vi "tcpcontrol.vi"() -> ()   [LabVIEW 2018]
uses:
  Downloads/sabertooth-packetized-control-master/sabertooth-packetized-control-master/code/package/controls/Sabertooth Baud Rate Select.ctl
  <vilib>/myRIO/Instrument Drivers/Onboard IO/DIO/typedefs/DIO Reference.ctl
  <vilib>/myRIO/Common/Instrument Driver Framework/Utilities/typedefs/myRIO Generic Hardware Reference.ctl
  <vilib>/myRIO/Common/Instrument Driver Framework/Utilities/typedefs/Hardware Version Enum.ctl
  <vilib>/myRIO/Common/Instrument Driver Framework/Utilities/typedefs/myRIO v1.0 Reference.ctl
  <vilib>/myRIO/Common/Instrument Driver Framework/Utilities/typedefs/Generic FPGA Reference.ctl
  <vilib>/myRIO/Common/Instrument Driver Framework/myRIO v1.0/DIO/typedefs/DIO Channels List.ctl
  <vilib>/myRIO/Common/Instrument Driver Framework/myRIO v1.0/DIO/typedefs/DIO Channels Enum.ctl
  <vilib>/userdefined/High Color/nirio_resource_hc.ctl
  <vilib>/myRIO/Common/Instrument Driver Framework/Utilities/vis/Is FPGA Ref Available.vi
  <vilib>/myRIO/Common/Instrument Driver Framework/myRIO v1.0/DIO/vis/myRIO v1.1 Open DIO.vi
  <vilib>/myRIO/Instrument Drivers/Onboard IO/DIO/vis/Write.vi
  <vilib>/myRIO/Common/Instrument Driver Framework/Utilities/vis/Validate Channels.vi
  <vilib>/myRIO/Common/Instrument Driver Framework/myRIO v1.0/DIO/vis/myRIO v1.0 Reserve DIO.vi
  <vilib>/myRIO/Common/Instrument Driver Framework/myRIO v1.0/Resource Manager/vis/myRIO v1.0 Reserve Channel List.vi
  <vilib>/myRIO/Common/Instrument Driver Framework/myRIO v1.0/DIO/vis/myRIO v1.0 Build MUX Configuration DIO.vi
  <vilib>/myRIO/Common/Instrument Driver Framework/myRIO v1.0/Resource Manager/vis/myRIO v1.0 Reserve Channel.vi
  <vilib>/myRIO/Common/Instrument Driver Framework/myRIO v1.0/Resource Manager/vis/myRIO v1.0 Unreserve Channel.vi
  <vilib>/myRIO/Common/Instrument Driver Framework/myRIO v1.0/Resource Manager/vis/myRIO v1.0 Create Configuration List.vi
  <vilib>/myRIO/Common/Instrument Driver Framework/myRIO v1.0/Resource Manager/vis/myRIO v1.0 Build Mutex Name.vi
  <vilib>/Instr/_visa.llb/VISA Configure Serial Port (Instr).vi
  <vilib>/Utility/VariantDataType/GetNumericInfo.vi
  <vilib>/Utility/error.llb/Error Cluster From Error Code.vi
  <vilib>/myRIO/Common/Instrument Driver Framework/myRIO v1.0/myRIO v1.1 Open.vi
  <vilib>/myRIO/Common/Instrument Driver Framework/Utilities/vis/IO Manager.vi
  <vilib>/myRIO/Common/Instrument Driver Framework/Utilities/vis/Configuration Manager.vi
  <vilib>/myRIO/Common/Instrument Driver Framework/myRIO v1.0/Resource Manager/vis/myRIO v1.0 Configure IO.vi
  <vilib>/myRIO/Common/Instrument Driver Framework/myRIO v1.0/myRIO v1.0 Close.vi
  <vilib>/myRIO/Common/Instrument Driver Framework/myRIO v1.0/DIO/vis/myRIO v1.0 Write DIO.vi
  <vilib>/myRIO/Express VI/Onboard Devices/LED/LED Express VI.xnode
  <vilib>/myRIO/Instrument Drivers/Onboard IO/DIO/vis/myRIO DIO Open.xnode
  <vilib>/myRIO/Instrument Drivers/Onboard IO/DIO/DIO.lvlib
panel:
  in  "stop 2":bool
  in  "Current Baud Rate":T1=115200 items=["2400 baud"=2400, "9600 baud"=9600, "19200 baud"=19200, "38400 baud"=38400, "115200 baud"=115200]
  in  "stop":bool
  out "Loop Time":u32
  out "error out":errorcluster
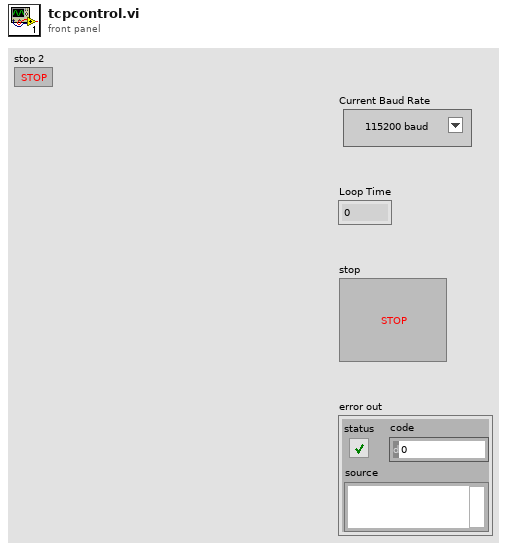
[diagram p1: front panel]
types:
  T1 = typedef "Sabertooth Baud Rate Select.ctl" = u32
  T2 = typedef "DIO.lvlib/DIO Reference.ctl" = cluster{"myRIO Reference":T3, "DIO Channels List":T7}
  T3 = typedef "myRIO Generic Hardware Reference.ctl" = cluster{"myRIO Model":T4, "myRIO Hardware Reference":T5}
  T4 = typedef "Hardware Version Enum.ctl" = enum16{"Unknown", "myRIO-1900", "myRIO-1950", "roboRIO", "NI ELVIS RIO CM", "ELVIS III"}
  T5 = typedef "myRIO v1.0 Reference.ctl" = cluster{"Generic FPGA Reference":T6, "Allow multiple opens":bool}
  T6 = typedef "Generic FPGA Reference.ctl" = refnum<k20>
  T7 = typedef "DIO Channels List.ctl" = T8[]
  T8 = typedef "DIO Channels Enum.ctl" = enum16{"Not Connected", "C/DIO0", "C/DIO1", "C/DIO2", "C/DIO3", "C/DIO4", "C/DIO5", "C/DIO6", "C/DIO7", "A/DIO0", "A/DIO1", "A/DIO2", "A/DIO3", "A/DIO4", "A/DIO5", "A/DIO6", "A/DIO7", "A/DIO8", "A/DIO9", "A/DIO10", "A/DIO11", "A/DIO12", "A/DIO13", "A/DIO14", "A/DIO15", "A/DIO16", "A/DIO17", "A/DIO18", "A/DIO19", "B/DIO0", "B/DIO1", "B/DIO2", "B/DIO3", "B/DIO4", "B/DIO5", "B/DIO6", "B/DIO7", "B/DIO8", "B/DIO9", "B/DIO10", "B/DIO11", "B/DIO12", "B/DIO13", "B/DIO14", "B/DIO15", "B/DIO16", "B/DIO17", "B/DIO18", "B/DIO19", "LED0", "LED1", "LED2", "LED3", "Button0", "DIO/DIO0", "DIO/DIO1", "DIO/DIO2", "DIO/DIO3", "DIO/DIO4", "DIO/DIO5", "DIO/DIO6", "DIO/DIO7", "DIO/DIO8", "DIO/DIO9", "SPI/CS0", "SPI/CS1", "SPI/CS2", "SPI/CS3", "LED RADIO (Green)", "LED RADIO (Red)", "LED COMM (Green)", "LED COMM (Red)", "LED MODE (Green)", "LED MODE (Red)"}
  T9 = typedef "nirio_resource_hc.ctl" = tag
  T10 = enum16{"Standard", "Buffered", "CRLF", "Immediate"}
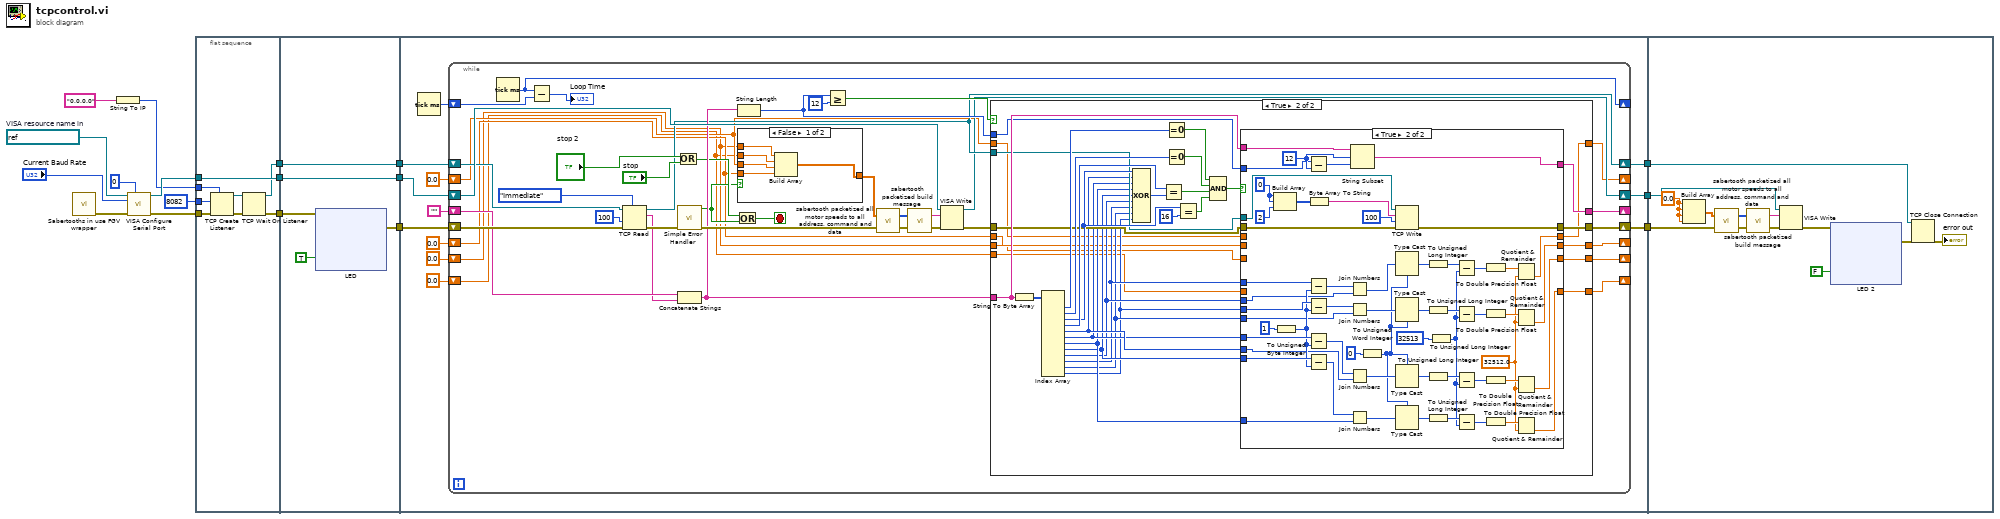
[diagram p0: block diagram]
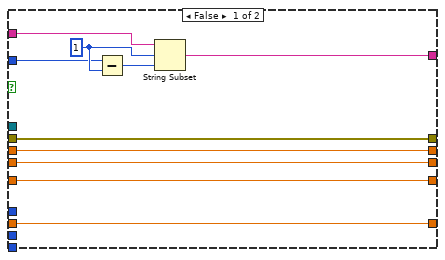
[diagram p3: hidden frame]
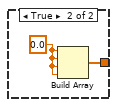
[diagram p4: hidden frame]
diagram:
  w18 = refnum<visa-resource-name> "ASRL1::INSTR"  # VISA resource name in
  n1 = call "Sabertooths in use FGV wrapper.vi"() -> ("error out"=w15:errorcluster)  [unwired: 11 in]
  n2 = String To IP(1:"0.0.0.0") -> (0:w12:u32)
  n3 = call-poly "VISA Configure Serial Port"("VISA resource name"=w18, "timeout (10sec)"=u32 0, "baud rate (9600)"="Current Baud Rate", "error in (no error)"=w15) -> ("VISA resource name out"=w17:refnum<visa-resource-name>, "error out"=w11:errorcluster)  [unwired: 10 in]
  n4 = flat-sequence {
    tunnel: w17 -> [w26]
    tunnel: [w26] -> w9
    tunnel: [w25] -> w7
    tunnel: [w24] -> w5
    tunnel: w12 -> [w23]
    tunnel: w11 -> [w22]
    tunnel: u16 8082 ("port") -> [w21]
    tunnel: w9 -> [w31]
    tunnel: [w31] -> w8
    tunnel: w7 -> [w29]
    tunnel: [w28] -> w6
    tunnel: w5 -> [w30]
    tunnel: [w30] -> w4
    tunnel: w8 -> [w78]
    tunnel: w6 -> [w76]
    tunnel: w4 -> [w75]
    tunnel: [w69] -> w3
    tunnel: [w68] -> w2
    tunnel: [w67] -> w1
    tunnel: w3 -> [w234]
    tunnel: w2 -> [w237]
    tunnel: w1 -> [w231]
    frame #0 {
      n5 = TCP Create Listener(7:w23, 8:w22, 10:w21) -> (0:w20:errorcluster, 3:w19:refnum<k5>)  [unwired: 2 in, 1 out]
      n6 = TCP Wait On Listener(8:w20, 11:w19) -> (0:w25:errorcluster, 3:w24:refnum<k5>)  [unwired: 2 in, 3 out]
    }
    frame #1 {
      n7 = xnode "LED"("LED0"=TRUE, "error in (no error)"=w29) -> ("error out"=w28:errorcluster)
    }
    frame #2 {
      n8 = Tick Count (ms)() -> (millisecond timer value=w77:u32)
      n9 = while {
        shift-right: [w114] -> _
        shift-left: w77 -> [w116]
        shift-right: [w90] -> w67
        shift-left: w75 -> [w107]
        shift-right: [w95] -> _
        shift-left: "" -> [w100]
        shift-right: [w86] -> _
        shift-left: 0.0 -> [w79]
        shift-right: [w85] -> _
        shift-left: 0.0 -> [w82]
        shift-right: [w84] -> _
        shift-left: 0.0 -> [w80]
        shift-right: [w83] -> _
        shift-left: 0.0 -> [w81]
        shift-right: [w88] -> w69
        shift-left: w76 -> [w106]
        shift-right: [w87] -> w68
        shift-left: w78 -> [w117]
        stop <- w92 stop-if-true
        n10 = Tick Count (ms)() -> (millisecond timer value=w114:u32)
        n11 = Subtract(x=w114, y=w116) -> (x-y=→"Loop Time":u32)
        n12 = TCP Read(connection ID=w107, error in (no error)=w106, 7:T10."Immediate" ("mode (standard)"), 9:100) -> (connection ID out=w90:refnum<k5>, data out=w99:string, error out=w104:errorcluster)  [unwired: 1 in]
        n13 = Or(x="stop 2", y="stop") -> (x .or. y?=w94:bool)
        n14 = call <vilib>:"Simple Error Handler.vi"("error in (no error)"=w104) -> ("error?"=w93:bool, "error out"=w103:errorcluster)  [unwired: 4 in, 3 out]
        n15 = Concatenate Strings(w100, w99) -> (w96:string)
        n16 = Or(x=w94, y=w93) -> (x .or. y?=w92:bool)
        n17 = String Length(string=w96) -> (length=w91:i32)
        n18 = case shown="False" w93 {
          tunnel: [w224 w229] -> w102
          tunnel: w80 -> [w228 _]
          tunnel: w79 -> [w227 _]
          tunnel: w81 -> [w226 _]
          tunnel: w82 -> [w225 _]
          frame False {
            n19 = Build Array(w228, w227, w226, w225) -> (w224:dbl[])
          }
          frame True {
            w230 = 0.0
            n20 = Build Array(w230, w230, w230, w230) -> (w229:dbl[])
          }
        }
        n21 = Greater Or Equal?(x=w91, y=12) -> (x >= y?=w97:bool)
        n22 = call "sabertooth packetized all motor speeds to all address, command and data.vi"("error in (no error)"=w103, "All Motor Speeds"=w102) -> ("error out"=w112:errorcluster, "Data to write"=w113:u8[][][])
        n23 = call "sabertooth packetized build message.vi"("error in (no error)"=w112, "Data to write"=w113) -> ("error out"=w111:errorcluster, "Uart Write Data"=w110:string)
        n24 = VISA Write(VISA resource name=w117, write buffer=w110, error in (no error)=w111) -> (VISA resource name out=w87:refnum<visa-resource-name>, error out=w89:errorcluster)  [unwired: 1 out]
        n25 = case shown="True" w97 {
          tunnel: w96 -> [w123 w145]
          tunnel: [w123 w144] -> w95
          tunnel: w91 -> [_ w143]
          tunnel: w90 -> [_ w142]
          tunnel: w89 -> [w122 w141]
          tunnel: [w122 w140] -> w88
          tunnel: [w118 w131] -> w86
          tunnel: [w121 w130] -> w85
          tunnel: [w119 w129] -> w84
          tunnel: [w120 w128] -> w83
          tunnel: w82 -> [w121 w127]
          tunnel: w81 -> [w120 w126]
          tunnel: w80 -> [w119 w125]
          tunnel: w79 -> [w118 w124]
          frame False {
          }
          frame True {
            n26 = String To Byte Array(string=w145) -> (unsigned byte array=w157:u8[])
            n27 = Index Array(array=w157) -> (element #1=w156:u8, element #2=w155:u8, element #3=w148:u8, element #4=w154:u8, element #5=w139:u8, element #6=w138:u8, element #7=w137:u8, element #8=w136:u8, element #9=w135:u8, element #10=w134:u8, element #11=w133:u8, element #12=w132:u8)  [unwired: 12 in]
            n28 = Compound Arithmetic op=XOR(w148, w139, w138, w137, w136, w135, w134, w133, w132) -> (w153:u8)
            n29 = Equal?(x=w154, y=w153) -> (x = y?=w150:bool)
            n30 = Equal To 0?(x=w156) -> (x = 0?=w152:bool)
            n31 = Equal To 0?(x=w155) -> (x = 0?=w151:bool)
            n32 = Equal?(x=w148, y=16) -> (x = y?=w149:bool)
            n33 = Compound Arithmetic op=AND(w152, w151, w150, w149) -> (w146:bool)
            n34 = case shown="True" w146 {
              tunnel: w145 -> [w164 w221]
              tunnel: [w163 w220] -> w144
              tunnel: w143 -> [w165 w219]
              tunnel: w142 -> [_ w212]
              tunnel: w141 -> [w162 w214]
              tunnel: [w162 w213] -> w140
              tunnel: w139 -> [_ w171]
              tunnel: w138 -> [_ w205]
              tunnel: w137 -> [_ w169]
              tunnel: w136 -> [_ w199]
              tunnel: w135 -> [_ w175]
              tunnel: w134 -> [_ w190]
              tunnel: w133 -> [_ w173]
              tunnel: w132 -> [_ w184]
              tunnel: [w158 w183] -> w131
              tunnel: [w161 w182] -> w130
              tunnel: [w159 w181] -> w129
              tunnel: [w160 w180] -> w128
              tunnel: w127 -> [w161 _]
              tunnel: w126 -> [w160 _]
              tunnel: w125 -> [w159 _]
              tunnel: w124 -> [w158 _]
              frame False {
                w166 = 1
                n35 = Subtract(x=w165, y=w166) -> (x-y=w167:i32)
                n36 = String Subset(string=w164, offset (0)=w166, length (rest)=w167) -> (substring=w163:string)
              }
              frame True {
                w176 = 32512.0
                w218 = 0
                w222 = 12
                n37 = Build Array(w218, w218, 2) -> (w216:i32[])
                n38 = To Unsigned Byte Integer(number=1) -> (unsigned 8bit integer=w178:u8)
                n39 = Subtract(x=w219, y=w222) -> (x-y=w223:i32)
                n40 = Subtract(x=w190, y=w178) -> (x-y=w174:u8)
                n41 = Subtract(x=w184, y=w178) -> (x-y=w172:u8)
                n42 = Subtract(x=w205, y=w178) -> (x-y=w170:u8)
                n43 = Subtract(x=w199, y=w178) -> (x-y=w168:u8)
                n44 = Byte Array To String(unsigned byte array=w216) -> (string=w215:string)
                n45 = Join Numbers(hi=w174, lo=w175) -> ((hi.lo)=w198:u16)
                n46 = Join Numbers(hi=w172, lo=w173) -> ((hi.lo)=w189:u16)
                n47 = Join Numbers(hi=w170, lo=w171) -> ((hi.lo)=w210:u16)
                n48 = Join Numbers(hi=w168, lo=w169) -> ((hi.lo)=w204:u16)
                n49 = String Subset(string=w221, offset (0)=w222, length (rest)=w223) -> (substring=w220:string)
                n50 = To Unsigned Word Integer(number=0) -> (unsigned 16bit integer=w179:u16)
                n51 = TCP Write(connection ID=w212, data in=w215, error in (no error)=w214, 9:100) -> (error out=w213:errorcluster)  [unwired: 2 out]
                n52 = Type Cast(type=w179, x=w198) -> (*(type *) &x=w195:u16)
                n53 = Type Cast(type=w179, x=w189) -> (*(type *) &x=w188:u16)
                n54 = Type Cast(type=w179, x=w210) -> (*(type *) &x=w209:u16)
                n55 = Type Cast(type=w179, x=w204) -> (*(type *) &x=w203:u16)
                n56 = To Unsigned Long Integer(number=w195) -> (unsigned 32bit integer=w194:u32)
                n57 = To Unsigned Long Integer(number=w188) -> (unsigned 32bit integer=w187:u32)
                n58 = To Unsigned Long Integer(number=w209) -> (unsigned 32bit integer=w208:u32)
                n59 = To Unsigned Long Integer(number=w203) -> (unsigned 32bit integer=w202:u32)
                n60 = To Unsigned Long Integer(number=32513) -> (unsigned 32bit integer=w177:u32)
                n61 = Subtract(x=w194, y=w177) -> (x-y=w191:u32)
                n62 = Subtract(x=w187, y=w177) -> (x-y=w185:u32)
                n63 = Subtract(x=w208, y=w177) -> (x-y=w206:u32)
                n64 = Subtract(x=w202, y=w177) -> (x-y=w200:u32)
                n65 = To Double Precision Float(number=w191) -> (double precision float=w192:dbl)
                n66 = To Double Precision Float(number=w185) -> (double precision float=w186:dbl)
                n67 = To Double Precision Float(number=w206) -> (double precision float=w207:dbl)
                n68 = To Double Precision Float(number=w200) -> (double precision float=w201:dbl)
                n69 = Quotient & Remainder(x=w192, y=w176) -> (floor(x/y)=w180:dbl)  [unwired: 1 out]
                n70 = Quotient & Remainder(x=w186, y=w176) -> (floor(x/y)=w182:dbl)  [unwired: 1 out]
                n71 = Quotient & Remainder(x=w207, y=w176) -> (floor(x/y)=w181:dbl)  [unwired: 1 out]
                n72 = Quotient & Remainder(x=w201, y=w176) -> (floor(x/y)=w183:dbl)  [unwired: 1 out]
              }
            }
          }
        }
      }
    }
    frame #3 {
      w236 = 0.0
      n73 = Build Array(w236, w236, w236, w236) -> (w235:dbl[])
      n74 = call "sabertooth packetized all motor speeds to all address, command and data.vi"("error in (no error)"=w234, "All Motor Speeds"=w235) -> ("error out"=w242:errorcluster, "Data to write"=w243:u8[][][])
      n75 = call "sabertooth packetized build message.vi"("error in (no error)"=w242, "Data to write"=w243) -> ("error out"=w241:errorcluster, "Uart Write Data"=w240:string)
      n76 = VISA Write(VISA resource name=w237, write buffer=w240, error in (no error)=w241) -> (error out=w238:errorcluster)  [unwired: 2 out]
      n77 = xnode "LED 2"("LED0"=FALSE, "error in (no error)"=w238) -> ("error out"=w233:errorcluster)
      n78 = TCP Close Connection(connection ID=w231, error in (no error)=w233) -> (error out=→"error out":errorcluster)  [unwired: 1 in, 1 out]
    }
  }
